vi "tx.vi"(8 "error in (no error)":errorcluster, 10 "tx":string, 11 "tcp server in":refnum<class "tcp connection.lvclass">) -> (0 "error out":errorcluster, 3 "tcp server out":refnum<class "tcp connection.lvclass">)   [LabVIEW 2014, in "tcp connection.lvclass"]
uses:
  tcp connection.lvclass
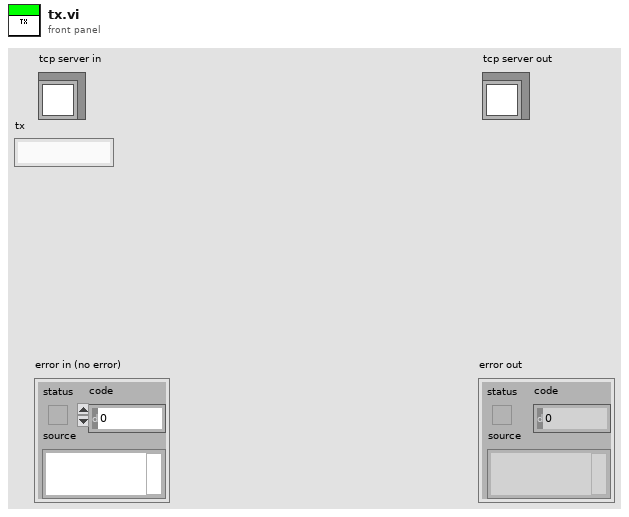
[diagram p1: front panel]
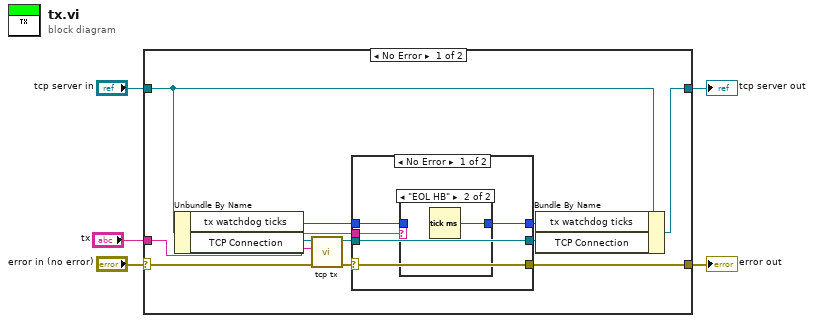
[diagram p0: block diagram]
diagram:
  n1 = case shown="No Error" "error in (no error)" {
    selector: "error in (no error)" -> [w10 w28]
    tunnel: [w16 w28] -> w4
    tunnel: [w14 w27] -> w2
    tunnel: "tcp server in" -> [w15 w27]
    tunnel: "tx" -> [w6 _]
    frame No Error {
      n2 = Unbundle By Name(w15) -> ("tx watchdog ticks"=w8:u32, "TCP Connection"=w12:refnum<k5>)
      n3 = call "tcp tx.vi"("error in"=w10, "tx"=w6, "TCP Connection in"=w12) -> ("error out"=w9:errorcluster, "TCP Connection out"=w11:refnum<k5>)  [unwired: 7 in]
      n4 = case shown="No Error" w9 {
        selector: w9 -> [w21 w24]
        tunnel: [w21 w24] -> w16
        tunnel: w11 -> [w20 w25]
        tunnel: [w20 w25] -> w13
        tunnel: w8 -> [w17 w26]
        tunnel: [w19 w26] -> w7
        tunnel: w6 -> [w18 _]
        frame No Error {
          n5 = case shown="\"EOL HB\"" w18 {
            tunnel: [w22 w23] -> w19
            tunnel: w17 -> [w22 _]
            frame Default {
            }
            frame "EOL HB" {
              n6 = Tick Count (ms)() -> (millisecond timer value=w23:u32)
            }
          }
        }
        frame Error {
        }
      }
      n7 = Bundle By Name(cluster=w15, "tx watchdog ticks"=w7, "TCP Connection"=w13) -> (w14:refnum<class "tcp connection.lvclass">)
    }
    frame Error {
    }
  }
  "error out" <- w4
  "tcp server out" <- w2
